vi "Inspect - Compute Transition Value.vi"(5 "Transition Criteria":T1 {"Function" items=["Equal"=0, "Not equal"=1, "Less"=2, "Less or Equal"=3, "Greater"=4, "Greater or Equal"=5, "In Range"=6, "Match Pattern"=7, "NaN"=8, "Result Not Available"=65535]; "Values"."Numeric Constant" format="%.2f"}) -> (2 "Transition Value":bool)   [LabVIEW 2019]
uses:
  Common.llb/IVB State Machine - Transitions Criteria.ctl
  Common.llb/IVB State Machine - Transitions Criteria Function.ctl
  Common.llb/IVB Result Data Types.ctl
  Common.llb/IVB State Machine - Transitions Criteria Result.ctl
  Common.llb/IVB Measure ID.ctl
panel:
  # "VI Name: Inspect - Compute Transition Value.vi\nPurpose: Evaluates a transition."
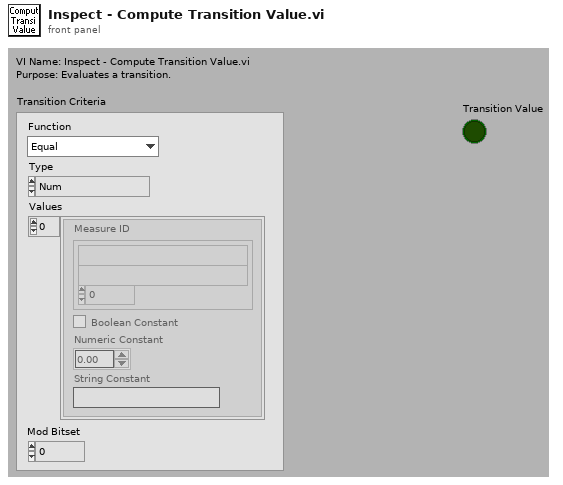
[diagram p1: front panel]
types:
  T1 = typedef "IVB State Machine - Transitions Criteria.ctl" = cluster{"Function":T2, "Type":T3, "Values":T4[], "Mod Bitset":i32}
  T2 = typedef "IVB State Machine - Transitions Criteria Function.ctl" = u16
  T3 = typedef "IVB Result Data Types.ctl" = enum16{"Num", "Bool", "Str", "1D Num", "1D Bool", "1D Str", "Pass/Fail"}
  T4 = typedef "IVB State Machine - Transitions Criteria Result.ctl" = cluster{"Measure ID":T5, "Boolean Constant":bool, "Numeric Constant":dbl, "String Constant":string}
  T5 = typedef "IVB Measure ID.ctl" = cluster{"Step GUID":string, "Result GUID":string, "Index":i32}
  T6 = cluster{"Numeric":dbl, "Boolean":bool, "String":string, "1D Numeric":dbl[], "1D Boolean":bool[], "1D String":string[]}
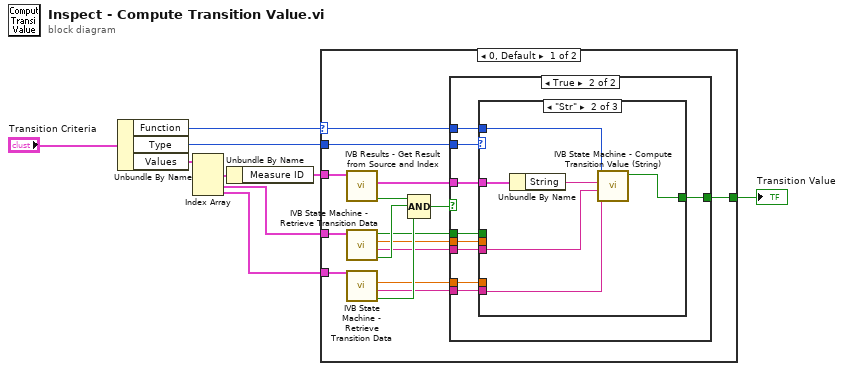
[diagram p0: block diagram]
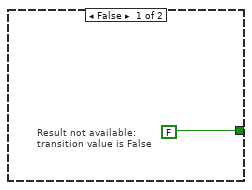
[diagram p2: hidden frame]
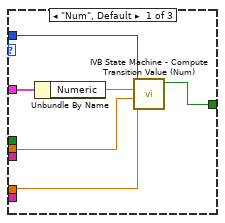
[diagram p3: hidden frame]
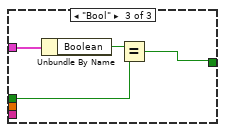
[diagram p4: hidden frame]
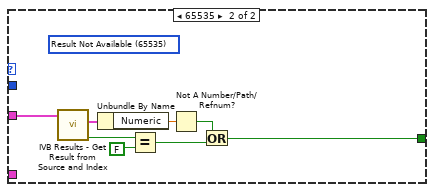
[diagram p5: hidden frame]
diagram:
  n1 = Unbundle By Name("Transition Criteria") -> ("Function"=w3:T2, "Type"=w4:T3, "Values"=w6:T4[])
  n2 = Index Array(array=w6) -> (element #1=w5:T4, element #2=w8:T4, element #3=w9:T4)  [unwired: 3 in]
  n3 = Unbundle By Name(w5) -> ("Measure ID"=w7:T5)
  n4 = case shown="0, Default" w3 {
    selector: w3 -> [w15 _]
    tunnel: [w24 w53] -> w1
    tunnel: w4 -> [w25 _]
    tunnel: w7 -> [w23 w52]
    tunnel: w8 -> [w22 _]
    tunnel: w9 -> [w21 _]
    frame 0, Default {
      n5 = call "IVB Results - Get Result from Source and Index.vi"("Measure ID"=w23) -> ("Result Available"=w20:bool, "Result Value"=w17:T6)  [unwired: 6 in, 3 out]
      n6 = call "IVB State Machine - Retrieve Transition Data.vi"("Transition Criteria Data"=w22) -> ("Result Available"=w19:bool, "String Value"=w11:string, "Numeric Value"=w13:dbl, "Boolean Value"=w14:bool)  [unwired: 7 in]
      n7 = call "IVB State Machine - Retrieve Transition Data.vi"("Transition Criteria Data"=w21) -> ("Result Available"=w18:bool, "String Value"=w10:string, "Numeric Value"=w12:dbl)  [unwired: 7 in, 1 out]
      n8 = Compound Arithmetic op=AND(w20, w19, w18) -> (w16:bool)
      n9 = case shown="True" w16 {
        tunnel: w25 -> [_ w35]
        tunnel: [FALSE w34] -> w24
        tunnel: w17 -> [_ w33]
        tunnel: w15 -> [_ w32]
        tunnel: w14 -> [_ w31]
        tunnel: w13 -> [_ w30]
        tunnel: w12 -> [_ w29]
        tunnel: w11 -> [_ w28]
        tunnel: w10 -> [_ w27]
        frame False {
          # "Result not available: transition value is False"
        }
        frame True {
          n10 = case shown="\"Str\"" w35 {
            tunnel: [w36 w45 w48] -> w34
            tunnel: w33 -> [w41 w47 w50]
            tunnel: w32 -> [w39 w46 _]
            tunnel: w31 -> [_ _ w49]
            tunnel: w30 -> [w38 _ _]
            tunnel: w29 -> [w37 _ _]
            tunnel: w28 -> [_ w43 _]
            tunnel: w27 -> [_ w42 _]
            frame "Num", Default {
              n11 = Unbundle By Name(w41) -> ("Numeric"=w40:dbl)
              n12 = call "IVB State Machine - Compute Transition Value (Num).vi"("Value 3"=w37, "Value 2"=w38, "Value 1"=w40, "Function"=w39) -> ("Transition Value"=w36:bool)  [unwired: 7 in]
            }
            frame "Str" {
              n13 = Unbundle By Name(w47) -> ("String"=w44:string)
              n14 = call "IVB State Machine - Compute Transition Value (String).vi"("Value 3"=w42, "Value 2"=w43, "Value 1"=w44, "Function"=w46) -> ("Transition Value"=w45:bool)  [unwired: 7 in]
            }
            frame "Bool" {
              n15 = Unbundle By Name(w50) -> ("Boolean"=w51:bool)
              n16 = Equal?(x=w51, y=w49) -> (x = y?=w48:bool)
            }
          }
        }
      }
    }
    frame 65535 {
      (unwired) T2 65535 items=["Equal"=0, "Not equal"=1, "Less"=2, "Less or Equal"=3, "Greater"=4, "Greater or Equal"=5, "In Range"=6, "Match Pattern"=7, "Result Not Available"=65535] ("Function")
      n17 = call "IVB Results - Get Result from Source and Index.vi"("Measure ID"=w52) -> ("Result Available"=w55:bool, "Result Value"=w54:T6)  [unwired: 6 in, 3 out]
      n18 = Unbundle By Name(w54) -> ("Numeric"=w58:dbl)
      n19 = Equal?(x=w55, y=FALSE) -> (x = y?=w57:bool)
      n20 = Not A Number/Path/Refnum?(number/path/refnum=w58) -> (NaN/Path/Refnum?=w59:bool)
      n21 = Or(x=w59, y=w57) -> (x .or. y?=w53:bool)
    }
  }
  "Transition Value" <- w1
